vi "Sum_Natural_Numbers.vi"() -> ()   [LabVIEW 2024]
panel:
  out "Input 2":dbl
  in  "Numeric":i32
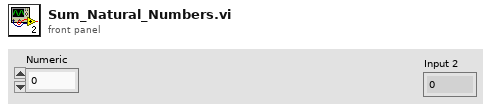
[diagram p1: front panel]
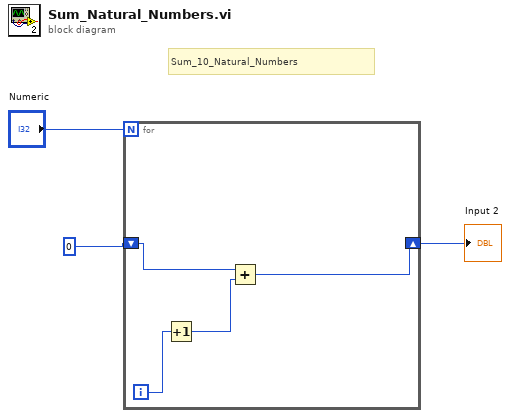
[diagram p0: block diagram]
diagram:
  # "Sum_10_Natural_Numbers"
  n1 = for {
    N: "Numeric" -> [_]
    shift-right: [w6] -> w2
    shift-left: 0 -> [w7]
    i -> [w5]
    n2 = Increment(x=w5) -> (x+1=w4:i32)
    n3 = Add(x=w7, y=w4) -> (x+y=w6:i32)
  }
  "Input 2" <- w2
